vi "Set Log File Specification.vi"(8 "error in (no error)":errorcluster, 10 "Log File Specification.lvclass":refnum<class "Log File Specification.lvclass">, 11 "Segmented Log in":refnum<class "Segmented Log.lvclass">) -> (0 "error out":errorcluster, 3 "Segmented Log out":refnum<class "Segmented Log.lvclass">)   [LabVIEW 2015, in "Segmented Log.lvclass"]
uses:
  Segmented Log.lvclass
  Log File Specifications/Log File Specification/Log File Specification.lvclass
  Segmented Log.lvclass/Segmented Log.ctl
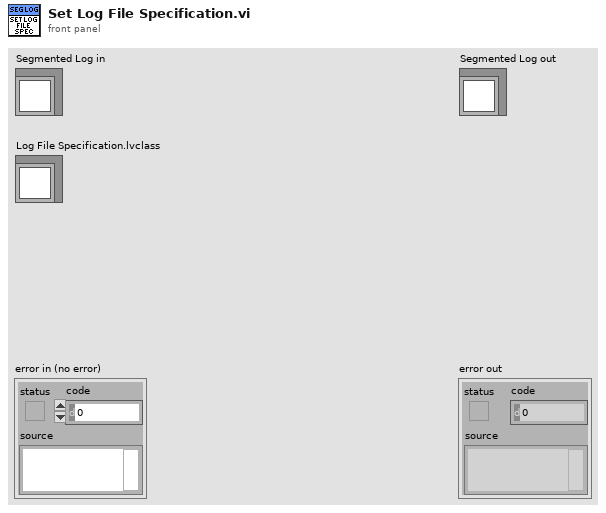
[diagram p1: front panel]
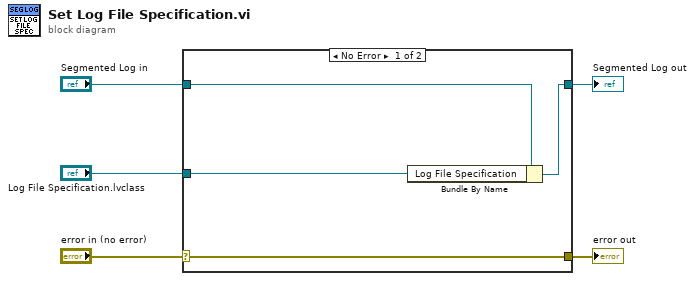
[diagram p0: block diagram]
diagram:
  n1 = case shown="No Error" "error in (no error)" {
    selector: "error in (no error)" -> [w9 w10]
    tunnel: [w9 w10] -> w4
    tunnel: [w7 w11] -> w2
    tunnel: "Segmented Log in" -> [w8 w11]
    tunnel: "Log File Specification.lvclass" -> [w6 _]
    frame No Error {
      n2 = Bundle By Name(cluster=w8, "Log File Specification"=w6) -> (w7:refnum<class "Segmented Log.lvclass">)
    }
    frame Error {
    }
  }
  "error out" <- w4
  "Segmented Log out" <- w2
